vi "move2zip.vi"(4 "error in":errorcluster, 6 "dest dir":path, 7 "source path":path) -> (0 "error out":errorcluster, 3 "zipped path":path)   [LabVIEW 2010]
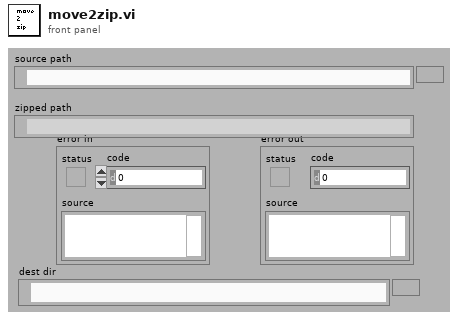
[diagram p1: front panel]
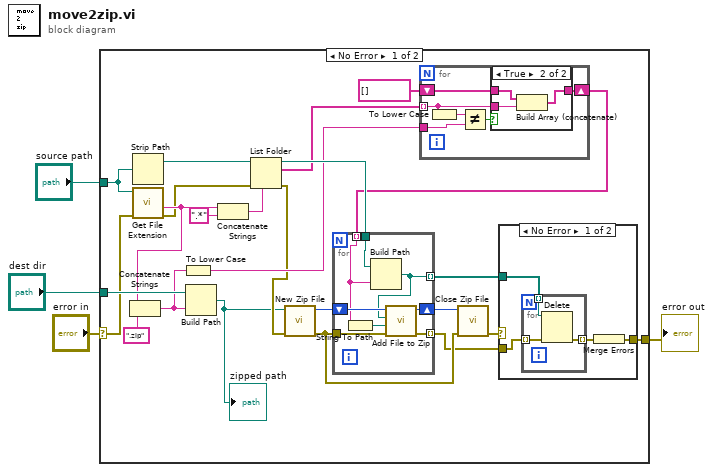
[diagram p0: block diagram]
diagram:
  n1 = case shown="No Error" "error in" {
    selector: "error in" -> [w13 w55]
    tunnel: [w26 w55] -> w4
    tunnel: "dest dir" -> [w25 _]
    tunnel: "source path" -> [w15 _]
    frame No Error {
      n2 = Strip Path(path=w15) -> (stripped path=w23:path)  [unwired: 1 out]
      n3 = call <vilib>:"Get File Extension.vi"("error in (no error)"=w13, "file"=w15) -> ("error out"=w12:errorcluster, "filename without extension"=w14:string)  [unwired: 6 in, 2 out]
      n4 = Concatenate Strings(w14, ".zip" ("replace string (\"\")")) -> (w10:string)
      n5 = To Lower Case(string=w10) -> (all lower case string=w9:string)
      n6 = Build Path(base path=w25, name or relative path=w10) -> (appended path=w5:path)
      "zipped path" <- w5
      n7 = Concatenate Strings(w14, ".*" ("string")) -> (w22:string)
      n8 = List Folder(path=w23, pattern=w22, error in=w12) -> (path out=w20:path, filenames=w11:string[], error out=w6:errorcluster)  [unwired: 1 in, 1 out]
      n9 = call <vilib>:"New Zip File.vi"("error in (no error)"=w6, "target"=w5) -> ("error out"=w18:errorcluster, "zip file out"=w27:i64)  [unwired: 3 in, 1 out]
      n10 = for {
        tunnel: w11 -> [w31] mode=indexing
        tunnel: w9 -> [w33]
        shift-right: [w30] -> w7
        shift-left: string[] [] -> [w29]
        n11 = To Lower Case(string=w31) -> (all lower case string=w34:string)
        n12 = Not Equal?(x=w34, y=w33) -> (x != y?=w32:bool)
        n13 = case shown="True" w32 {
          tunnel: w31 -> [_ w38]
          tunnel: [w35 w37] -> w30
          tunnel: w29 -> [w35 w36]
          frame False {
          }
          frame True {
            n14 = Build Array (concatenate)(w36, w38) -> (w37:string[])
          }
        }
      }
      n15 = for {
        tunnel: [w45] -> w17 mode=indexing
        tunnel: w18 -> [w43]
        tunnel: w20 -> [w42]
        tunnel: w7 -> [w40] mode=indexing
        tunnel: [w39] -> w19 mode=indexing
        shift-right: [w46] -> w28
        shift-left: w27 -> [w44]
        n16 = String To Path(string=w40) -> (path=w41:path)
        n17 = Build Path(base path=w42, name or relative path=w40) -> (appended path=w39:path)
        n18 = call <vilib>:"Add File to Zip.vi"("error in (no error)"=w43, "destination path in zip"=w41, "source file path"=w39, "zip file in"=w44) -> ("error out"=w45:errorcluster, "zip file out"=w46:i64)  [unwired: 6 in]
      }
      n19 = call <vilib>:"Close Zip File.vi"("error in (no error)"=w18, "zip file in"=w28) -> ("error out"=w16:errorcluster)  [unwired: 5 in]
      n20 = case shown="No Error" w16 {
        selector: w16 -> [_ w54]
        tunnel: w19 -> [w50 _]
        tunnel: [w47 w54] -> w26
        tunnel: w17 -> [w49 _]
        frame No Error {
          n21 = for {
            tunnel: w50 -> [w53] mode=indexing
            tunnel: [w52] -> w48 mode=indexing
            tunnel: w49 -> [w51] mode=indexing
            n22 = Delete(path (use dialog)=w53, error in=w51) -> (error out=w52:errorcluster)  [unwired: 3 in, 2 out]
          }
          n23 = Merge Errors(w48) -> (w47:errorcluster)
        }
        frame Error {
        }
      }
    }
    frame Error {
    }
  }
  "error out" <- w4
